vi "Apply Override File.vi"(8 "error in (no error)":errorcluster, 10 "Override File Path":path, 11 "System Definition Path in":path) -> (0 "error out":errorcluster, 3 "System Definition Path out":path)   [LabVIEW 2020]
uses:
  niveristand-custom-device-testing-tools/VeriStandTestUtilities/VeriStandTestUtilities.lvlib
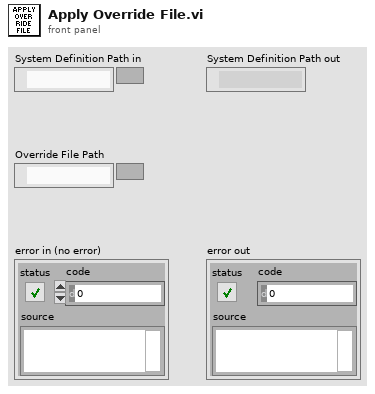
[diagram p1: front panel]
types:
  T1 = typedef "VeriStandTestUtilities.lvlib/ConfigOverrideItem.ctl" = cluster{"node":string, "property":string, "value":string}
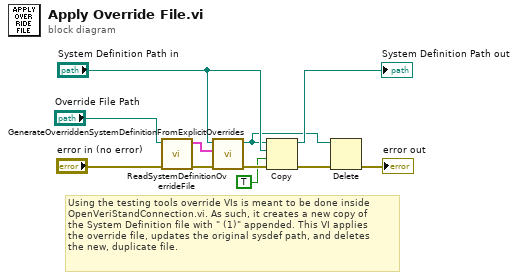
[diagram p0: block diagram]
diagram:
  # "Using the testing tools override VIs is meant to be done inside\nOpenVeriStandConnection.vi. As such, it creates a new copy of\nthe System Definition file with \" (1)\" appended. This VI applies\nthe override file, updates the original sysdef path, and deletes\nthe new, duplicate file."
  n1 = call "ReadSystemDefinitionOverrideFile.vi"("error in (no error)"="error in (no error)", "configuration file path"="Override File Path") -> ("error out"=w10:errorcluster, "overrides"=w11:T1[])  [unwired: 7 in, 1 out]
  n2 = call "GenerateOverriddenSystemDefinitionFromExplicitOverrides.vi"("error in (no error)"=w10, "overrides"=w11, "absolute system definition file"="System Definition Path in") -> ("error out"=w7:errorcluster, "absolute overridden system definition file"=w2:path)  [unwired: 6 in, 1 out]
  n3 = Copy(8:w7, 9:TRUE ("overwrite (F)"), 10:"System Definition Path in", 11:w2) -> (0:w4:errorcluster, 3:→"System Definition Path out":path)  [unwired: 1 in, 1 out]
  n4 = Delete(path (use dialog)=w2, error in=w4) -> (error out=→"error out":errorcluster)  [unwired: 3 in, 2 out]
